vi "FTW-Logger-Destroy.vi"(0 "FTW Logger":refnum<class "FTW-Logger-Core.lvclass">, 11 "error in":errorcluster) -> (15 "error out":errorcluster)   [LabVIEW 2013, in "FTW-Logger-Core.lvclass"]
uses:
  FTW-Logger-Core.lvclass
  FTW-Logger-Core.lvclass/FTW-Logger-Core.ctl
panel:
  # "Inputs"
  # "Outputs"
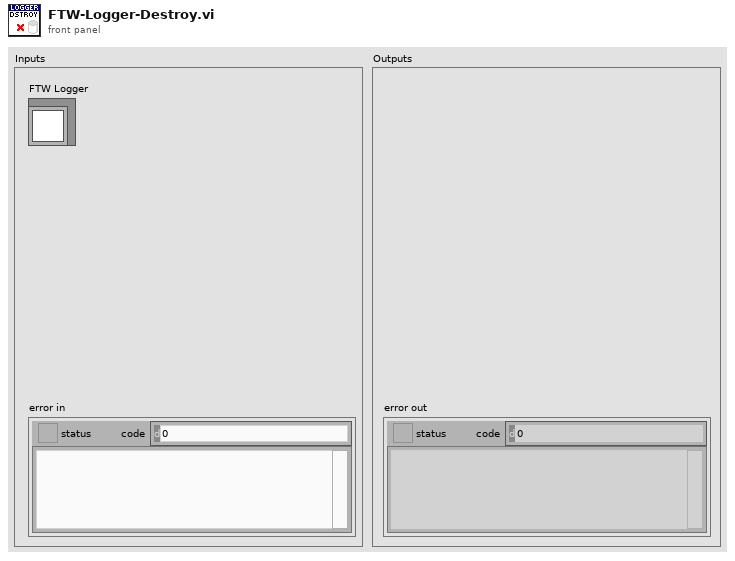
[diagram p1: front panel]
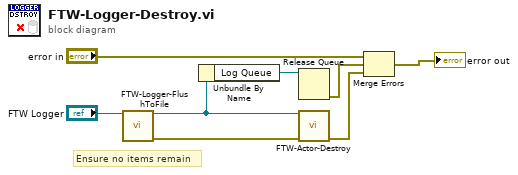
[diagram p0: block diagram]
diagram:
  # "Ensure no items remain"
  n1 = call "FTW-Logger-FlushToFile.vi"("FTW Logger"="FTW Logger") -> ("FTW Logger out"=w2:refnum<class "FTW-Logger-Core.lvclass">, "error out"=w5:errorcluster)  [unwired: 13 in]
  n2 = Unbundle By Name(w2) -> ("Log Queue"=w3:refnum<queue>)
  n3 = Release Queue(queue=w3) -> (error out=w1:errorcluster)  [unwired: 2 in, 2 out]
  n4 = call-dynamic "FTW-Actor-Destroy.vi"("FTW Actor Instance"=w2, "error in"=w5) -> ("error out"=w4:errorcluster)  [unwired: 13 in]
  n5 = Merge Errors("error in", w1, w4) -> (→"error out":errorcluster)
